vi "New Card Setup 2.vi"(0 "Generic Instrument in":refnum<class "Generic Instrument.lvclass">, 5 "Card Array":bool[](array[boolean]), 11 "error in (no error)":errorcluster) -> (4 "Generic Instrument out":refnum<class "Generic Instrument.lvclass">, 6 "decimal integer string":string[](array[string]), 8 "Continuous?":bool, 10 "Card chosen":i32, 14 "Time Cluster":T1, 15 "error out":errorcluster)   [LabVIEW 2013, in "Generic Instrument.lvlib" / "Generic Instrument.lvclass"]
uses:
  Generic Instrument.lvclass
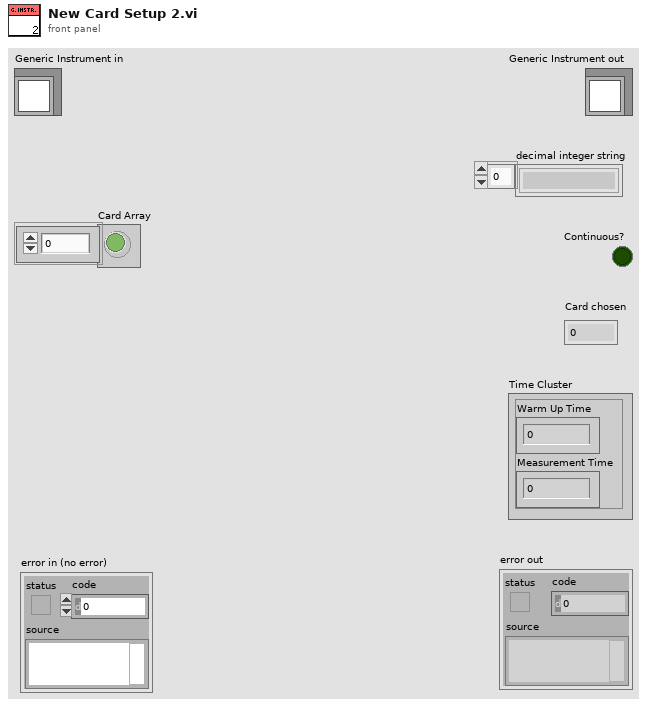
[diagram p1: front panel]
types:
  T1 = cluster{"Warm Up Time":dbl, "Measurement Time":dbl}
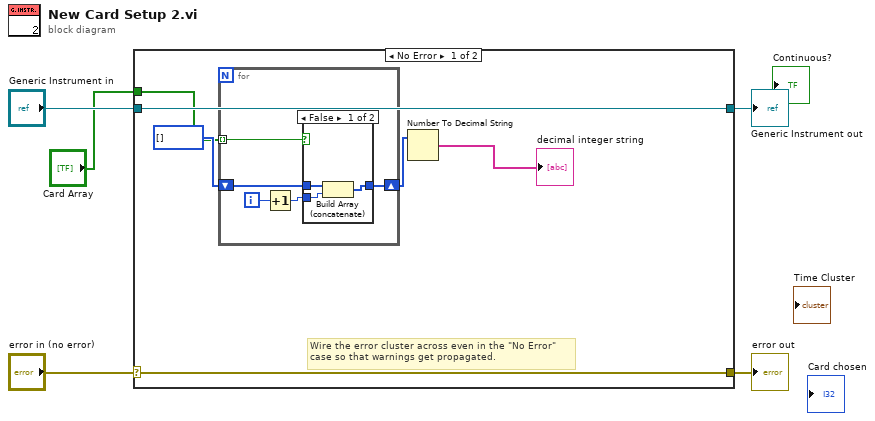
[diagram p0: block diagram]
diagram:
  n1 = case shown="No Error" "error in (no error)" {
    selector: "error in (no error)" -> [w10 w22]
    tunnel: [w10 w22] -> w4
    tunnel: [w11 w21] -> w2
    tunnel: "Generic Instrument in" -> [w11 w21]
    tunnel: "Card Array" -> [w6 _]
    frame No Error {
      # "Wire the error cluster across even in the \"No Error\"\ncase so that warnings get propagated."
      n2 = for {
        tunnel: w6 -> [w16] mode=indexing
        shift-right: [w12] -> w8
        shift-left: i32[] [] -> [w15]
        i -> [w14]
        n3 = Increment(x=w14) -> (x+1=w13:i32)
        n4 = case shown="False" w16 {
          tunnel: w15 -> [w19 w20]
          tunnel: w13 -> [w18 _]
          tunnel: [w17 w20] -> w12
          frame False {
            n5 = Build Array (concatenate)(w19, w18) -> (w17:i32[])
          }
          frame True {
          }
        }
      }
      n6 = Number To Decimal String(number=w8) -> (decimal integer string=→"decimal integer string":string[])  [unwired: 1 in]
    }
    frame Error {
    }
  }
  "error out" <- w4
  "Generic Instrument out" <- w2
